vi "Configure Marker Function.vi"(7 "Marker Function":T1, 8 "error in (no error)":errorcluster, 10 "Marker Number (1)":u32=1 min=1, 11 "MXA in":refnum<class "MXA.lvclass">) -> (0 "error out":errorcluster, 3 "MXA out":refnum<class "MXA.lvclass">)   [LabVIEW 2020, in "MXA.lvclass"]
uses:
  MXA.lvclass
  C:/Sandbox/Git_Sandbox/WiSpry Test Framework source code (LV20)/WiSpry Test Framework/Instruments/Instrument.lvclass
  Controls/Marker Functions.ctl
  Instrument.lvclass/Instrument.ctl
  Instrument.lvclass
  <instrlib>/Agilent MXA Series/Agilent MXA Series.lvlib
  Spectrum Analyzer.lvclass
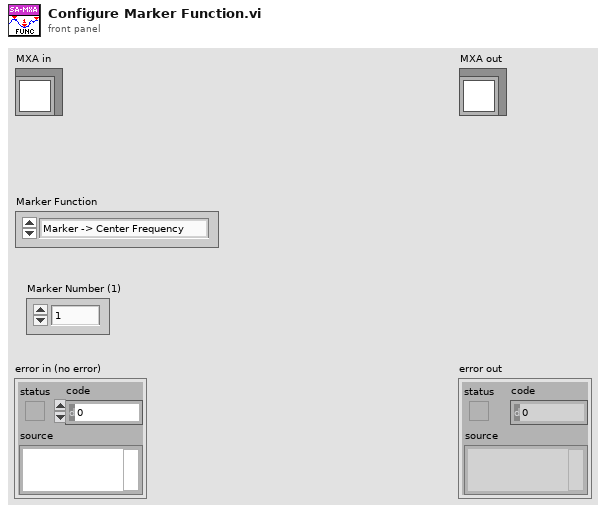
[diagram p1: front panel]
types:
  T1 = typedef "Spectrum Analyzer.lvclass/Marker Functions.ctl" = enum16{"Marker -> Center Frequency", "Marker -> Reference Level"}
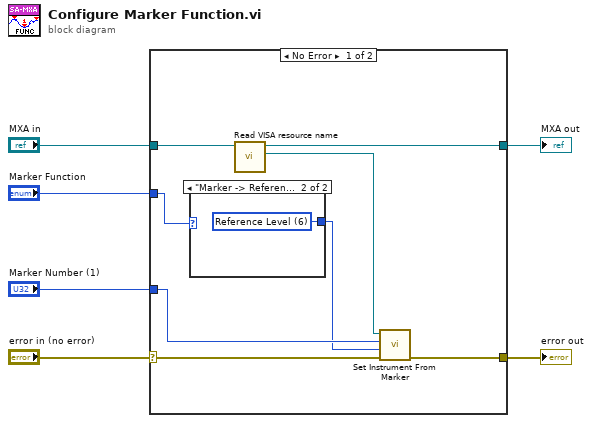
[diagram p0: block diagram]
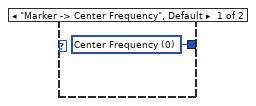
[diagram p2: hidden frame]
diagram:
  n1 = case shown="No Error" "error in (no error)" {
    selector: "error in (no error)" -> [w11 w18]
    tunnel: "MXA in" -> [w14 w17]
    tunnel: [w10 w18] -> w5
    tunnel: [w13 w17] -> w4
    tunnel: "Marker Number (1)" -> [w9 _]
    tunnel: "Marker Function" -> [w8 _]
    frame No Error {
      n2 = case shown="\"Marker -> Reference Level\"" w8 {
        tunnel: [w15 w16] -> w7
        frame "Marker -> Center Frequency", Default {
          w15 = 0 items=["Center Frequency", "Center Frequency Step", "Start Frequency", "Stop Frequency", "Delta Span", "Delta Center Frequency", "Reference Level"] ("Instrument Setting (0: Center Frequency)")
        }
        frame "Marker -> Reference Level" {
          w16 = 6 items=["Center Frequency", "Center Frequency Step", "Start Frequency", "Stop Frequency", "Delta Span", "Delta Center Frequency", "Reference Level"] ("Instrument Setting (0: Center Frequency)")
        }
      }
      n3 = call "Read VISA resource name.vi"("Instrument in"=w14) -> ("VISA resource name"=w12:refnum<visa-resource-name>, "Instrument out"=w13:refnum<class "MXA.lvclass">)  [unwired: 9 in]
      n4 = call <instrlib>:"Set Instrument From Marker.vi"("error in (no error)"=w11, "Instrument Setting (0: Center Frequency)"=w7, "Active Marker (1: Marker1)"=w9, "VISA resource name"=w12) -> ("error out"=w10:errorcluster)  [unwired: 6 in, 1 out]
    }
    frame Error {
    }
  }
  "error out" <- w5
  "MXA out" <- w4
